vi "SmartSEM Remote API FIB Gun Valve.vi"(5 "Wait (ms)":u32=2000, 7 "Iterations":u32=3, 8 "error in":errorcluster, 10 "FIB Gun Valve":enum16{"Close", "Open"}(ring), 11 "ActiveX Container":refnum<k7>(container)) -> (0 "error out":errorcluster, 3 "reference out":refnum<k7>)   [LabVIEW 2018]
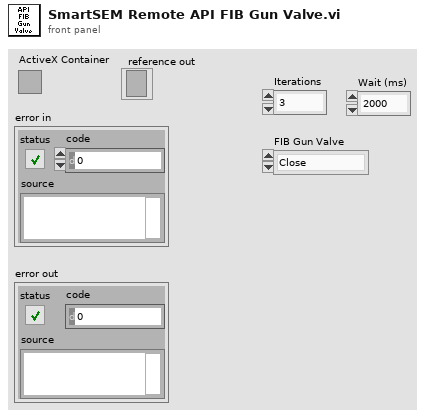
[diagram p1: front panel]
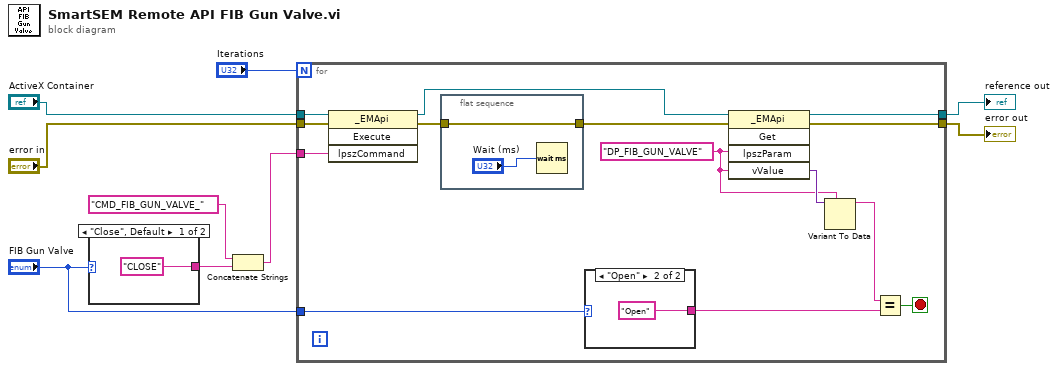
[diagram p0: block diagram]
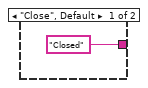
[diagram p2: hidden frame]
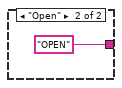
[diagram p3: hidden frame]
diagram:
  n1 = case shown="\"Close\", Default" "FIB Gun Valve" {
    tunnel: ["CLOSE" ("lpszCommand") "OPEN" ("lpszCommand")] -> w8
    frame "Close", Default {
    }
    frame "Open" {
    }
  }
  n2 = Concatenate Strings("CMD_FIB_GUN_VALVE_" ("lpszCommand"), w8) -> (w7:string)
  n3 = for {
    N: "Iterations" -> [_]
    tunnel: "ActiveX Container" -> [w25]
    tunnel: w7 -> [w24]
    tunnel: "FIB Gun Valve" -> [w12]
    tunnel: "error in" -> [w20]
    tunnel: [w19] -> w4
    tunnel: [w18] -> w5
    stop <- w21 stop-if-true
    w15 = "DP_FIB_GUN_VALVE" ("lpszParam")
    n4 = invoke class="_EMApi" method="Execute"(reference=w25, error in=w20, "lpszCommand"=w24) -> (reference out=w23:refnum<k7>, error out=w17:errorcluster)  [unwired: 1 in, 2 out]
    n5 = flat-sequence {
      tunnel: [w29] -> w16
      tunnel: w17 -> [w29]
      frame #0 {
        n6 = Wait (ms)(milliseconds to wait="Wait (ms)") -> ()  [unwired: 1 out]
      }
    }
    n7 = case shown="\"Open\"" w12 {
      tunnel: ["Closed" ("lpszCommand") "Open" ("lpszCommand")] -> w14
      frame "Close", Default {
      }
      frame "Open" {
      }
    }
    n8 = invoke class="_EMApi" method="Get"(reference=w23, error in=w16, "lpszParam"=w15, "vValue"=w15) -> (reference out=w19:refnum<k7>, error out=w18:errorcluster, "vValue"=w22:variant)  [unwired: 1 in, 2 out]
    n9 = Variant To Data(type=w15, Variant=w22) -> (data=w13:string)  [unwired: 1 in, 1 out]
    n10 = Equal?(x=w13, y=w14) -> (x = y?=w21:bool)
  }
  "error out" <- w5
  "reference out" <- w4
